vi "decodeString.vi"(8 "error in (no error)":errorcluster, 11 "ByteArray":u8[](array[numeric]) format="%x") -> (0 "error out":errorcluster, 1 "String":string, 2 "Variant":variant, 3 "RemainingBytes":u8[](array[numeric]) format="%x", 5 "Type":string)   [LabVIEW 2015, in "MsgPack.lvlib"]
uses:
  MsgPack.lvlib
  <vilib>/ErrorRing/Error Ring.xnode
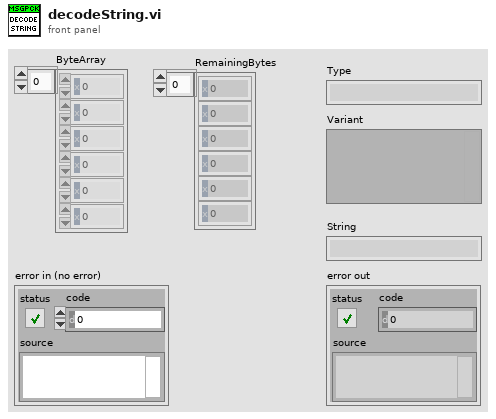
[diagram p1: front panel]
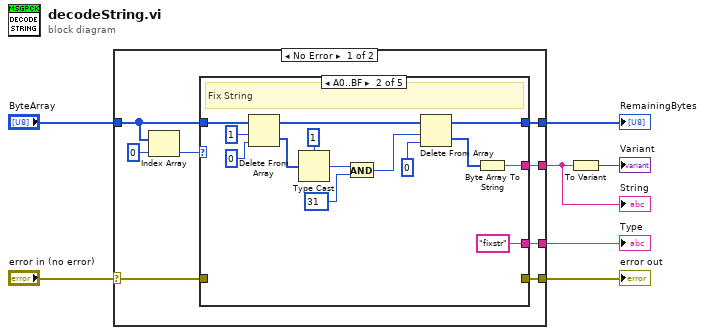
[diagram p0: block diagram]
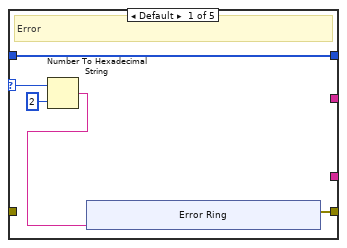
[diagram p2: hidden frame]
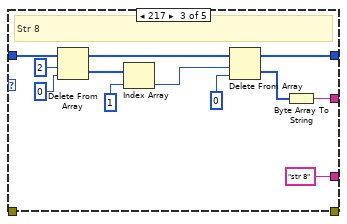
[diagram p3: hidden frame]
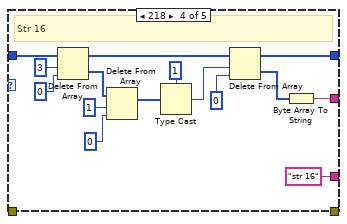
[diagram p4: hidden frame]
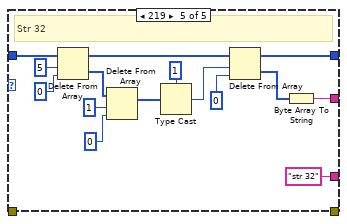
[diagram p5: hidden frame]
diagram:
  n1 = case shown="No Error" "error in (no error)" {
    selector: "error in (no error)" -> [w12 w83]
    tunnel: [w15 w83] -> w6
    tunnel: [w14 _] -> w5
    tunnel: [w13 _] -> w4
    tunnel: "ByteArray" -> [w10 w82]
    tunnel: [w11 w82] -> w2
    frame No Error {
      n2 = Index Array(array=w10, index=0) -> (element=w9:u8)
      n3 = case shown="A0..BF" w9 {
        selector: w9 -> [w17 _ _ _ _]
        tunnel: [w19 _ _ _ _] -> w15
        tunnel: w12 -> [_ _ _ _ _]
        tunnel: [_ "fixstr" "str 8" "str 16" "str 32"] -> w14
        tunnel: [_ w35 w47 w62 w77] -> w13
        tunnel: [w20 w27 w44 w58 w73] -> w11
        tunnel: w10 -> [w20 w37 w49 w64 w79]
        frame Default {
          # "Error"
          n4 = Number To Hexadecimal String(1:i16 2 ("width (-)"), 2:w17) -> (0:w16:string)
          n5 = xnode "Error Ring"("parameter 0"=w16) -> ("error out"=w19:errorcluster)
        }
        frame 160..191 {
          # "Fix String"
          n6 = Delete From Array(array=w37, length=1, index=0) -> (deleted portion=w32:u8[], array with subset deleted=w28:u8[])
          n7 = Type Cast(type=u8 1 ("index"), x=w32) -> (*(type *) &x=w30:u8)
          n8 = And(x=w30, y=u8 31) -> (x .and. y?=w33:u8)
          n9 = Delete From Array(array=w28, length=w33, index=0) -> (deleted portion=w26:u8[], array with subset deleted=w27:u8[])
          n10 = Byte Array To String(unsigned byte array=w26) -> (string=w35:string)
        }
        frame 217 {
          # "Str 8"
          n11 = Delete From Array(array=w49, length=2, index=0) -> (deleted portion=w42:u8[], array with subset deleted=w45:u8[])
          n12 = Index Array(array=w42, index=1) -> (element=w40:u8)
          n13 = Delete From Array(array=w45, length=w40, index=0) -> (deleted portion=w43:u8[], array with subset deleted=w44:u8[])
          n14 = Byte Array To String(unsigned byte array=w43) -> (string=w47:string)
        }
        frame 218 {
          # "Str 16"
          n15 = Delete From Array(array=w64, length=3, index=0) -> (deleted portion=w55:u8[], array with subset deleted=w59:u8[])
          n16 = Delete From Array(array=w55, length=1, index=0) -> (array with subset deleted=w54:u8[])  [unwired: 1 out]
          n17 = Type Cast(type=u16 1 ("index"), x=w54) -> (*(type *) &x=w56:u16)
          n18 = Delete From Array(array=w59, length=w56, index=0) -> (deleted portion=w57:u8[], array with subset deleted=w58:u8[])
          n19 = Byte Array To String(unsigned byte array=w57) -> (string=w62:string)
        }
        frame 219 {
          # "Str 32"
          n20 = Delete From Array(array=w79, length=5, index=0) -> (deleted portion=w70:u8[], array with subset deleted=w74:u8[])
          n21 = Delete From Array(array=w70, length=1, index=0) -> (array with subset deleted=w69:u8[])  [unwired: 1 out]
          n22 = Type Cast(type=u32 1 ("index"), x=w69) -> (*(type *) &x=w71:u32)
          n23 = Delete From Array(array=w74, length=w71, index=0) -> (deleted portion=w72:u8[], array with subset deleted=w73:u8[])
          n24 = Byte Array To String(unsigned byte array=w72) -> (string=w77:string)
        }
      }
    }
    frame Error {
    }
  }
  "error out" <- w6
  "Type" <- w5
  "String" <- w4
  "RemainingBytes" <- w2
  n25 = To Variant(anything=w4) -> (Variant=→"Variant":variant)
